vi "Shake Tray Impl.vi"(8 "error in (no error)":errorcluster, 10 "Time (s)":dbl=1.0, 11 "Simulated Autosampler in":refnum<class "Simulated Autosampler.lvclass">) -> (0 "error out":errorcluster, 3 "Simulated Autosampler out":refnum<class "Simulated Autosampler.lvclass">)   [LabVIEW 2023, in "Simulated Autosampler.lvlib" / "Simulated Autosampler.lvclass"]
uses:
  Simulated Autosampler.lvclass
  C:/FLASH/Development/Hardware/Autosampler/Autosampler.lvclass
  Autosampler/Autosampler State.ctl
  Simulated Autosampler.lvclass/Simulated Autosampler.ctl
  Autosampler/Autosampler.lvlib
  Autosampler/Autosampler.lvclass
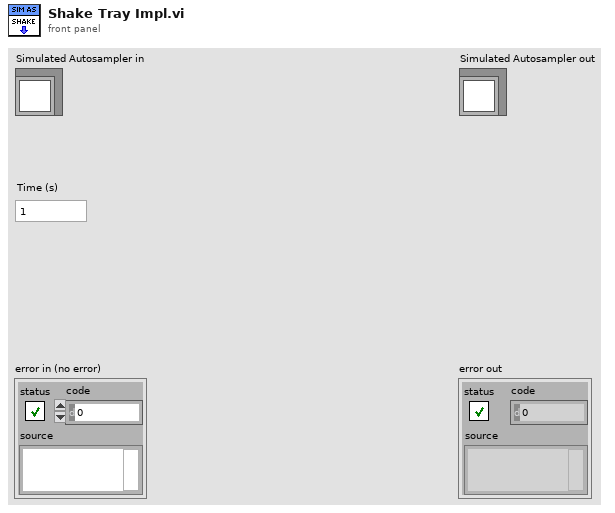
[diagram p1: front panel]
types:
  T1 = typedef "Autosampler.lvlib/Autosampler State.ctl" = enum16{"Ready", "Injection", "Washing", "Shaking", "Getting Ready", "Error"}
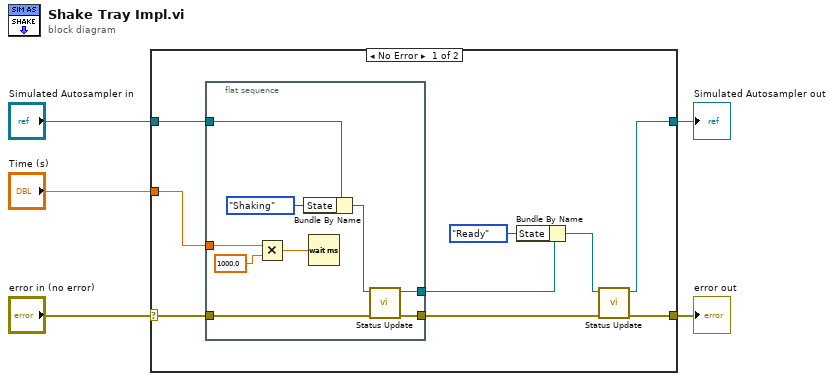
[diagram p0: block diagram]
diagram:
  n1 = case shown="No Error" "error in (no error)" {
    selector: "error in (no error)" -> [w8 w24]
    tunnel: [w6 w24] -> w4
    tunnel: "Simulated Autosampler in" -> [w10 w25]
    tunnel: [w7 w25] -> w2
    tunnel: "Time (s)" -> [w9 _]
    frame No Error {
      n2 = flat-sequence {
        tunnel: w10 -> [w21]
        tunnel: w8 -> [w23]
        tunnel: [w20] -> w12
        tunnel: [w22] -> w11
        tunnel: w9 -> [w17]
        frame #0 {
          n3 = Multiply(x=w17, y=1000.0) -> (x*y=w16:dbl)
          n4 = Bundle By Name(cluster=w21, "State"=Autosampler_State."Shaking" ("Autosampler Status.State")) -> (w19:refnum<class "Simulated Autosampler.lvclass">)
          n5 = Wait (ms)(milliseconds to wait=w16) -> ()  [unwired: 1 out]
          n6 = call "Status Update.vi"("error in (no error)"=w23, "Autosampler in"=w19) -> ("error out"=w22:errorcluster, "Autosampler out"=w20:refnum<class "Simulated Autosampler.lvclass">)  [unwired: 7 in, 1 out]
        }
      }
      n7 = Bundle By Name(cluster=w12, "State"=Autosampler_State."Ready" ("Autosampler Status.State")) -> (w13:refnum<class "Simulated Autosampler.lvclass">)
      n8 = call "Status Update.vi"("error in (no error)"=w11, "Autosampler in"=w13) -> ("error out"=w6:errorcluster, "Autosampler out"=w7:refnum<class "Simulated Autosampler.lvclass">)  [unwired: 7 in, 1 out]
    }
    frame Error {
    }
  }
  "error out" <- w4
  "Simulated Autosampler out" <- w2
